vi "Sub_Set_Voltage_List_SweepOutput.vi"(2 "error in (no error)":errorcluster, 3 "i":i32=1, 4 "AgB29xxLib.IAgB29xx2":refnum<k7>) -> (0 "error out":errorcluster, 1 "AgB29xxLib.IAgB29xx2 2":refnum<k7>)   [LabVIEW 2009]
panel:
  # "Sub VI: Set Voltage List Sweep Output"
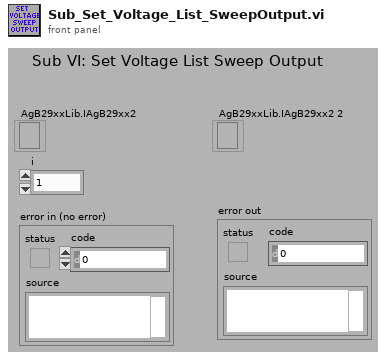
[diagram p1: front panel]
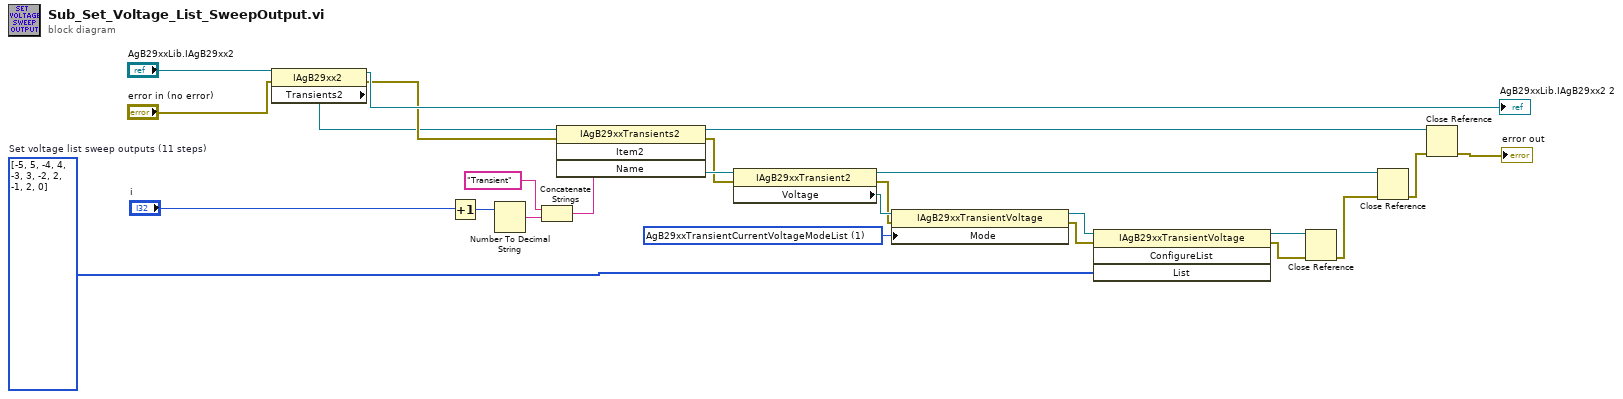
[diagram p0: block diagram]
diagram:
  w7 = 1 items=["AgB29xxTransientCurrentVoltageModeFixed", "AgB29xxTransientCurrentVoltageModeList", "AgB29xxTransientCurrentVoltageModeSweep"] ("Mode")
  w24 = i32[] [-5, 5, -4, 4, -3, 3, -2, 2, -1, 2, 0]  # Set voltage list sweep outputs (11 steps)
  n1 = property class="IAgB29xx2"(reference="AgB29xxLib.IAgB29xx2", error in="error in (no error)") -> (reference out=→"AgB29xxLib.IAgB29xx2 2":refnum<k7>, error out=w20:errorcluster, "Transients2"=w19:refnum<k7>)
  n2 = Increment(x="i") -> (x+1=w17:i32)
  n3 = Number To Decimal String(number=w17) -> (decimal integer string=w16:string)  [unwired: 1 in]
  n4 = Concatenate Strings("Transient" ("string"), w16) -> (w14:string)
  n5 = invoke class="IAgB29xxTransients2" method="Item2"(reference=w19, error in=w20, "Name"=w14) -> (reference out=w10:refnum<k7>, error out=w13:errorcluster, "Item2"=w18:refnum<k7>)  [unwired: 1 in, 1 out]
  n6 = property class="IAgB29xxTransient2"(reference=w18, error in=w13) -> (reference out=w12:refnum<k7>, error out=w8:errorcluster, "Voltage"=w9:refnum<k7>)
  n7 = property class="IAgB29xxTransientVoltage"(reference=w9, error in=w8, "Mode"=w7) -> (reference out=w6:refnum<k7>, error out=w5:errorcluster)
  n8 = invoke class="IAgB29xxTransientVoltage" method="ConfigureList"(reference=w6, error in=w5, "List"=w24) -> (reference out=w3:refnum<k7>, error out=w4:errorcluster)  [unwired: 1 in, 2 out]
  n9 = Close Reference(reference=w3, error in (no error)=w4) -> (error out=w2:errorcluster)
  n10 = Close Reference(reference=w12, error in (no error)=w2) -> (error out=w11:errorcluster)
  n11 = Close Reference(reference=w10, error in (no error)=w11) -> (error out=→"error out":errorcluster)
